vi "WiiMote Interface.vi"() -> ()   [LabVIEW 2017]
doc: "Uses the General Histogram VI to implement a running histogram.\n\nThis example generates continuous Gaussian noise, computes the histogram of the noise, and adds the new histogram to the sum of all the previous histograms.\n\nIn addition to computing the histogram, the General Histogram VI also computes the number of points that are outside all bins. This example keeps a running total of this quantity. The bins of the histogram span three standard deviations of the noise level.\n\nThe histogram plot should begin to resemble a Gaussian curve as more points are added to the histogram. The units of the histogram display are % of total points. \n\nNote: You must have the LabVIEW Full or Professional Development Systems to run this example. Also note that there is now a Point by Point function palette which provides an easier way to implement a running histogram. See the example Moving Histogram PtByPt.vi."
uses:
  C:/Users/rkr/EmbeddedLab_v1.70_Courseware-Kobuki/EmbeddedLab_v1.70_Courseware/Courseware/src/LabVIEW/WiiMote/Dependencies/WiimoteLib.dll
  Dependencies/WiimoteLib.dll
  <vilib>/Analysis/coordinate.llb/Angle Units.ctl
  <vilib>/Analysis/coordinate.llb/Wrap Angle (array).vi
  <vilib>/imath/engines/lvmath2/RunTimeEngine/IndexRead/NIMS V(S).vi
  <instcachedir>/0/NIMS V(S)_0488751826AF41519A22953C041130DC.lvgen/NIMS V(S)_0488751826AF41519A22953C041130DC_003.vi
  <vilib>/imathl/engines/lvmath/Functions/Error Handling/Create Error.vi
  <vilib>/imath/engines/lvmath2/RunTimeEngine/NodeEndStatement/NIMS_NodeEndStatement_Output.vi
  <instcachedir>/0/NIMS_NodeEndStatement_Output_53EC0D466D134D7ABD903AC30B43404B.lvgen/NIMS_NodeEndStatement_Output_53EC0D466D134D7ABD903AC30B43404B_013.vi
  <instcachedir>/0/NIMS_NodeEndStatement_Output_53EC0D466D134D7ABD903AC30B43404B.lvgen/NIMS_NodeEndStatement_Output_53EC0D466D134D7ABD903AC30B43404B_012.vi
  <instcachedir>/0/NIMS_NodeEndStatement_Output_53EC0D466D134D7ABD903AC30B43404B.lvgen/NIMS_NodeEndStatement_Output_53EC0D466D134D7ABD903AC30B43404B_011.vi
  <vilib>/imath/engines/lvmath2/RunTimeEngine/ErrorHandling/NIMS_Finalize Error.vi
  <instcachedir>/0/NIMS_NodeEndStatement_Output_53EC0D466D134D7ABD903AC30B43404B.lvgen/NIMS_NodeEndStatement_Output_53EC0D466D134D7ABD903AC30B43404B_010.vi
  <vilib>/Analysis/NI_AAL_Angle.lvlib
panel:
  in  "calibration (raw)":cluster{"bias":i32, "sensitivity":i32}={"bias"=0, "sensitivity"=29}
  out "Orientation (calibrated)":cluster{"Angle Out[0]":dbl, "Angle Out[1]":dbl}(graph)
  out "magnitude (g)":dbl
  out "Acceleration (calibrated)":cluster{"a[0]":i16, "a[1]":i16, "a[2]":i16}(graph)
  out "Acceleration (uncalibrated)":cluster{"X":sgl, "Y":sgl, "Z":sgl}(graph)
  in  "HID Transmit":u8=82 format="%02x"
  in  "measure sensitivity":bool
  in  "measure bias":bool caption="Record x-axis d0"
  in  "Payload":u8 format="%02x"
  in  "Report ID":u8 format="%02x"
  in  "Transmit":bool
  in  "stop":bool
  # "Part 3"
  # "Part 6 & 8"
  # "x"
  # "x"
  # "y"
  # "y"
  # "z"
  # "z"
  # "Calibration"
  # "Transmission"
  # "Part 7"
  # "Measure"
  # "roll"
  # "Set correctly for Part 5 of the lab."
  # "pitch"
  # "Set correctly for Part 4 of the lab. Be sure you can turn the vibration on and off."
  # "Stops the program, start is the arrow on the toolbars."
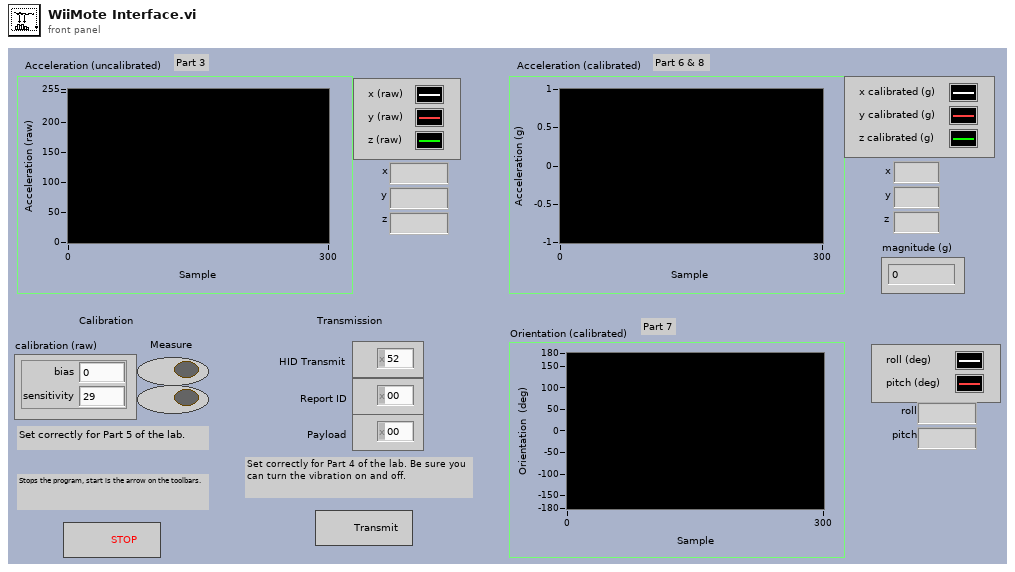
[diagram p1: front panel]
types:
  T1 = typedef "WiiMote State.ctl" = cluster{"X":sgl, "Y":sgl, "Z":sgl, "A":bool, "B":bool, "Down":bool, "Home":bool, "Left":bool, "Minus":bool, "One":bool, "Plus":bool, "Right":bool, "Two":bool, "Up":bool, "error out":errorcluster}
  T2 = typedef "NI_AAL_Angle.lvlib/Angle Units.ctl" = i32
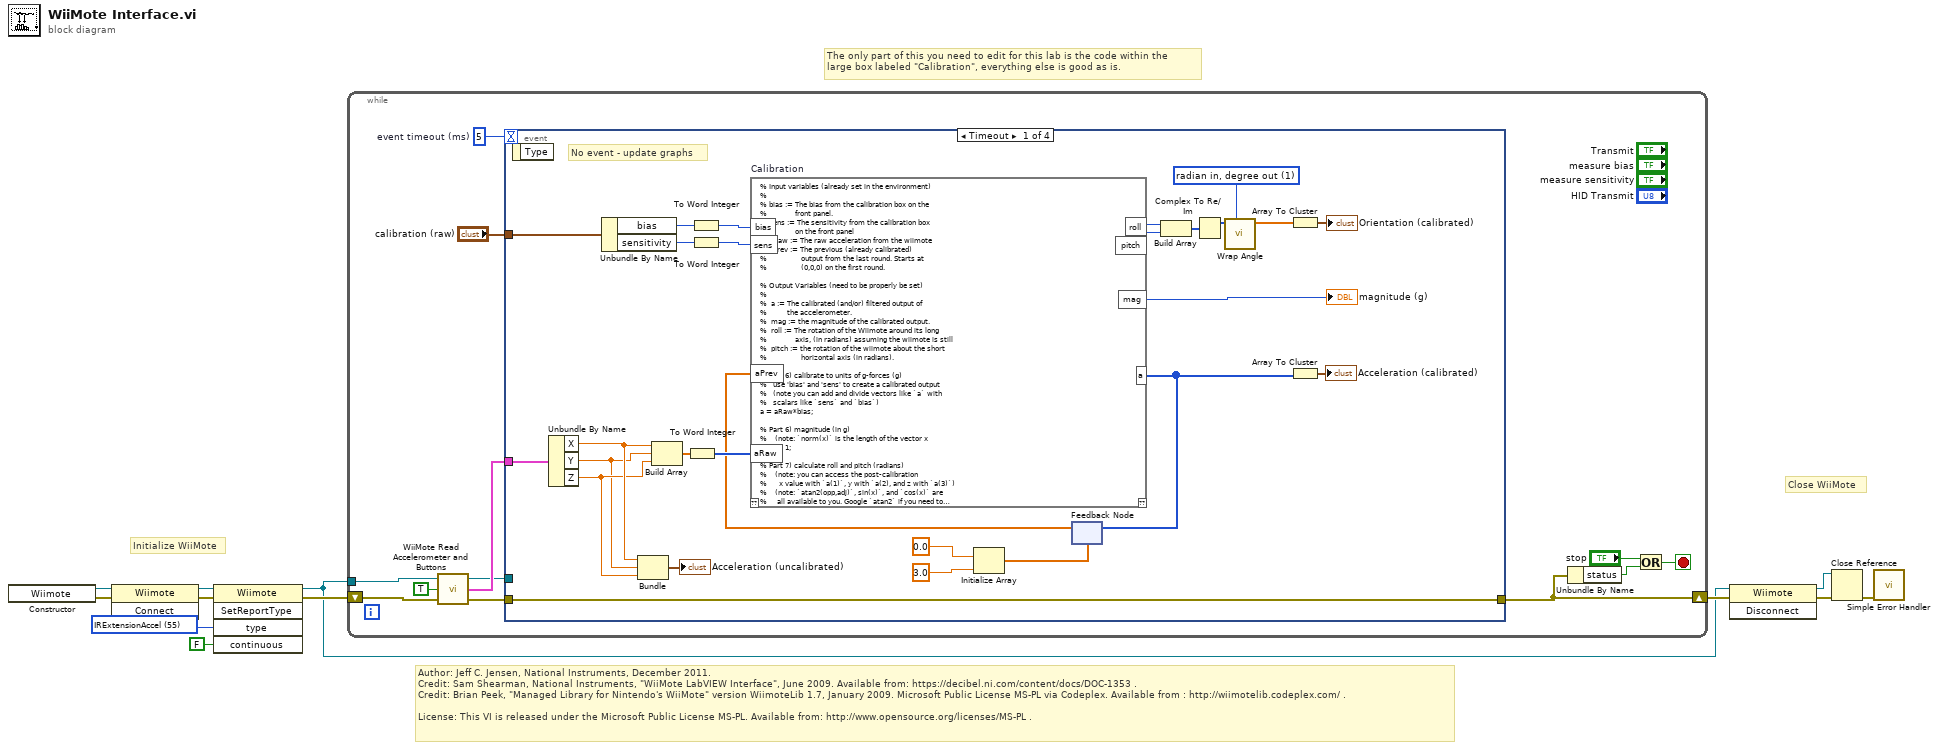
[diagram p0: block diagram]
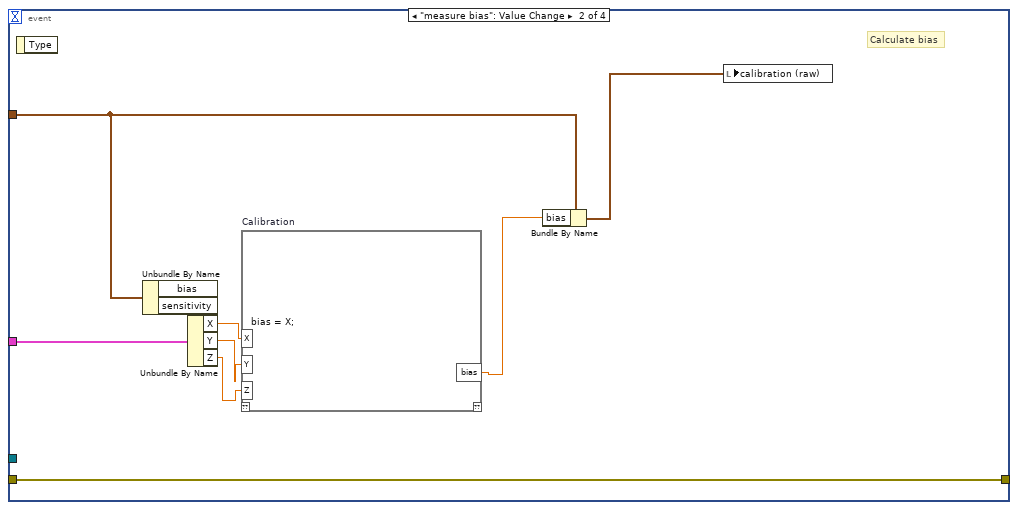
[diagram p2: hidden frame]
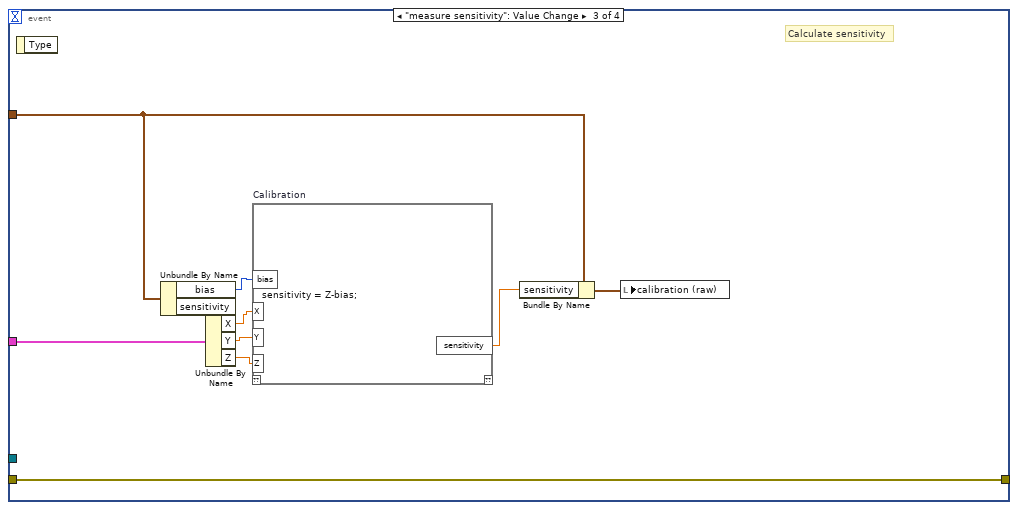
[diagram p3: hidden frame]
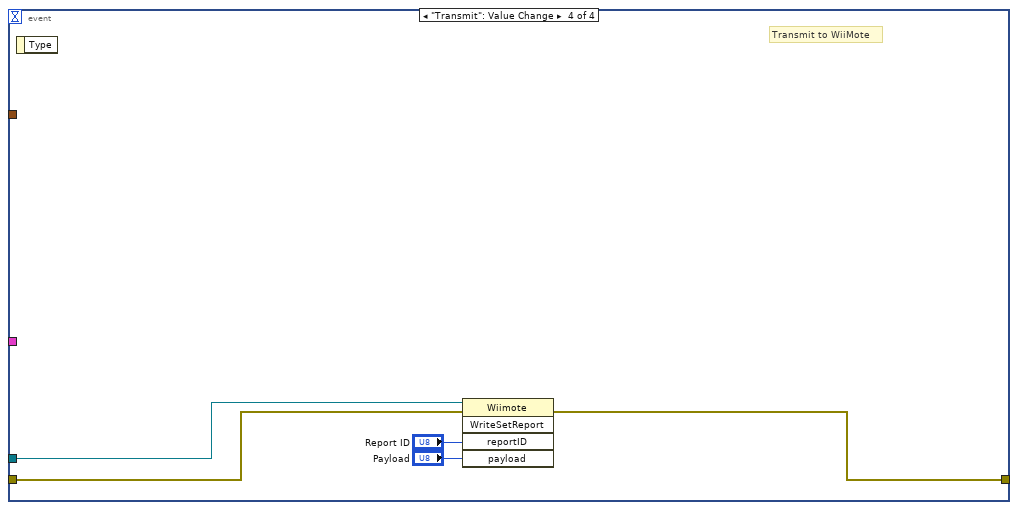
[diagram p4: hidden frame]
diagram:
  w10 = u8 55 items=["Status"=32, "ReadData"=33, "OutputReportAck"=34, "Buttons"=48, "ButtonsAccel"=49, "IRAccel"=51, "ButtonsExtension"=52, "ExtensionAccel"=53, "IRExtensionAccel"=55] ("type")
  # "The only part of this you need to edit for this lab is the code within the \nlarge box labeled \"Calibration\", everything else is good as is."
  # "Author: Jeff C. Jensen, National Instruments, December 2011.\nCredit: Sam Shearman, National Instruments, \"WiiMote LabVIEW Interface\", June 2009. Available from: https://decibel.ni.com/content/docs/DOC-1353 .\nCredit: Brian Peek, \"Managed Library for Nintendo's WiiMote\" version WiimoteLib 1.7, January 2009. Microsoft Public License MS-PL via Codeplex. Available from : http://wiimotelib.codeplex.com/ .\n\nLicense: This VI is released under the Microsoft Public License MS-PL. Available from: http://www.opensource.org/licenses/MS-PL ."
  # "Close WiiMote"
  # "Initialize WiiMote"
  n1 = constructor class="Wiimote"() -> (reference out=w11:refnum<k24>, error out=w12:errorcluster)  [unwired: 3 in, 1 out]
  n2 = invoke class="Wiimote" method="Connect"(reference=w11, error in=w12) -> (reference out=w1:refnum<k24>, error out=w8:errorcluster)  [unwired: 1 in, 1 out]
  n3 = invoke class="Wiimote" method="SetReportType"(reference=w1, error in=w8, "type"=w10, "continuous"=FALSE) -> (reference out=w3:refnum<k24>, error out=w7:errorcluster)  [unwired: 1 in, 3 out]
  n4 = while {
    tunnel: w3 -> [w23]
    shift-right: [w17] -> w9
    shift-left: w7 -> [w22]
    stop <- w24 stop-if-true
    w21 = 5  # event timeout (ms)
    n5 = call "WiiMote Read Accelerometer and Buttons.vi"("error in"=w22, "read raw values"=TRUE, "Wiimote"=w23) -> ("error out"=w19:errorcluster, "Wiimote State"=w20:T1, "reference out"=w18:refnum<k24>)
    n6 = event shown="[0] Timeout" {
      selector: _ -> [_ _ _ _]
      dyn-events: _ -> [_ _ _ _]
      timeout: w21 -> [_ _ _ _]
      tunnel: w20 -> [w51 w135 w162 _]
      tunnel: w19 -> [w50 w136 w161 w186]
      tunnel: w18 -> [_ _ _ w185]
      tunnel: [w50 w136 w161 w184] -> w17
      tunnel: "calibration (raw)" -> [w46 w133 w160 _]
      event Timeout {
        w31 = T2 1 items=["radian in, radian out", "radian in, degree out", "degree in, degree out", "degree in, radian out"] ("angle units")
        # "No event - update graphs"
        n7 = event-data() -> ()  [unwired: 1 in, 1 out]
        n8 = Unbundle By Name(w51) -> ("X"=w45:sgl, "Y"=w43:sgl, "Z"=w44:sgl)
        n9 = Unbundle By Name(w46) -> ("bias"=w48:i32, "sensitivity"=w47:i32)
        n10 = Bundle("X"=w45, "Y"=w43, "Z"=w44) -> (→"Acceleration (uncalibrated)":cluster{"X":sgl, "Y":sgl, "Z":sgl})  [unwired: 1 in]
        n11 = Build Array(w45, w43, w44) -> (w42:sgl[])
        n12 = To Word Integer(number=w42) -> (16bit integer=w39:i16[])
        n13 = To Word Integer(number=w48) -> (16bit integer=w41:i16)
        n14 = To Word Integer(number=w47) -> (16bit integer=w40:i16)
        n15 = Initialize Array(0.0, 3.0) -> (w25:dbl[])
        n16 = feedback #1(w25) -> (w28:dbl[])
        n17 = mathscript code="% Input variables (already set in the environment)\n%\n% bias := The bias from the calibration box on the\n%              front panel.\n% sens := The sensitivity from the calibration box \n%              on the front panel\n% aRaw := The raw acceleration from the wiimote\n% aPrev := The previous (already calibrated) \n%                 output from the last round. Starts at\n%                 (0,0,0) on the first round.\n\n% Output Variables (need to be properly be set)\n%\n%  a := The calibrated (and/or) filtered output of \n%          the accelerometer.\n%  mag := the magnitude of the calibrated output.\n%  roll := The rotation of the Wiimote around its long \n%              axis, (in radians) assuming the wiimote is still\n%  pitch := the rotation of the wiimote about the short\n%                 horizontal axis (in radians).\n\n% Part 6) calibrate to units of g-forces (g)\n%   use 'bias' and 'sens' to create a calibrated output\n%   (note you can add and divide vectors like `a` with\n%   scalars like `sens` and `bias`)\na = aRaw*bias;\n\n% Part 6) magnitude (in g)\n%    (note: `norm(x)` is the length of the vector x\nmag = 1;\n\n% Part 7) calculate roll and pitch (radians)\n%    (note: you can access the post-calibration\n%      x value with `a(1)`, y with `a(2), and z with `a(3)`)\n%    (note: `atan2(opp,adj)`, sin(x)`, and `cos(x)` are\n%     all available to you. Google `atan2` if you need to\n%     know more)\n%    (note: look at section 4 of the tilt compensated \n%       e-compass page, use Figure 1 on page 3 to find\n%       what the variables in the eqs mean)\nroll = a(1);\npitch =  a(3);\n\n% Part 8) Use `aPrev` and the algorithm from section 7.2\n%  of the 'Tilt compensated e-compass' article to create\n%  a low pass filter. \na = a;" "Calibration"("bias"=w41, "sens"=w40, "aRaw"=w39, "aPrev"=w28) -> ("mag"=→"magnitude (g)":i32, "a"=w29:i16[], "roll"=w34:i16, "pitch"=w33:i16)  [unwired: 1 in, 1 out]
        n18 = feedback-in #1(w29) -> ()
        n19 = Build Array(w34, w33) -> (w38:i16[])
        n20 = Complex To Re/Im(x + iy=w38) -> (x=w32:i16[])  [unwired: 1 out]
        n21 = call-poly <vilib>:"Wrap Angle.vi"("angle units"=w31, "Angle In"=w32) -> ("Angle Out"=w30:dbl[])  [unwired: 8 in, 1 out]
        n22 = Array To Cluster(array=w30) -> (cluster=→"Orientation (calibrated)":cluster{"Angle Out[0]":dbl, "Angle Out[1]":dbl})
        n23 = Array To Cluster(array=w29) -> (cluster=→"Acceleration (calibrated)":cluster{"a[0]":i16, "a[1]":i16, "a[2]":i16})
      }
      event "measure bias": Value Change {
        # "Calculate bias"
        n24 = event-data() -> ()  [unwired: 1 in, 1 out]
        n25 = Unbundle By Name(w133) -> ()  [unwired: 2 out]
        n26 = Unbundle By Name(w135) -> ("X"=w132:sgl, "Y"=w131:sgl, "Z"=w130:sgl)
        n27 = mathscript code="bias = X;" "Calibration"("X"=w132, "Y"=w131, "Z"=w130) -> ("bias"=w129:sgl)  [unwired: 1 in, 1 out]
        n28 = Bundle By Name(cluster=w133, "bias"=w129) -> (w134:cluster{"bias":i32, "sensitivity":i32})
        n29 = local write "calibration (raw)"(w134) -> ()
      }
      event "measure sensitivity": Value Change {
        # "Calculate sensitivity"
        n30 = event-data() -> ()  [unwired: 1 in, 1 out]
        n31 = Unbundle By Name(w160) -> ("bias"=w155:i32)  [unwired: 1 out]
        n32 = Unbundle By Name(w162) -> ("X"=w158:sgl, "Y"=w157:sgl, "Z"=w156:sgl)
        n33 = mathscript code="sensitivity = Z-bias;" "Calibration"("X"=w158, "Y"=w157, "Z"=w156, "bias"=w155) -> ("sensitivity"=w154:sgl)  [unwired: 1 in, 1 out]
        n34 = Bundle By Name(cluster=w160, "sensitivity"=w154) -> (w159:cluster{"bias":i32, "sensitivity":i32})
        n35 = local write "calibration (raw)"(w159) -> ()
      }
      event "Transmit": Value Change {
        # "Transmit to WiiMote"
        n36 = event-data() -> ()  [unwired: 1 in, 1 out]
        n37 = invoke class="Wiimote" method="WriteSetReport"(reference=w185, error in=w186, "reportID"="Report ID", "payload"="Payload") -> (error out=w184:errorcluster)  [unwired: 1 in, 4 out]
      }
    }
    n38 = Unbundle By Name(w17) -> ("status"=w15:bool)
    n39 = Or(x="stop", y=w15) -> (x .or. y?=w24:bool)
  }
  n40 = invoke class="Wiimote" method="Disconnect"(reference=w3, error in=w9) -> (reference out=w6:refnum<k24>, error out=w5:errorcluster)  [unwired: 1 in, 1 out]
  n41 = Close Reference(reference=w6, error in (no error)=w5) -> (error out=w4:errorcluster)
  n42 = call <vilib>:"Simple Error Handler.vi"("error in (no error)"=w4) -> ()  [unwired: 4 in, 5 out]
